vi "ENPH 354 Assignment 2 - Q3 .vi"() -> ()   [LabVIEW 2021]
panel:
  out "Top Right":bool
  out "Top":bool
  out "Top Left":bool
  out "Middle":bool
  out "Bottom Right":bool
  out "Bottom Left":bool
  out "Bottom":bool
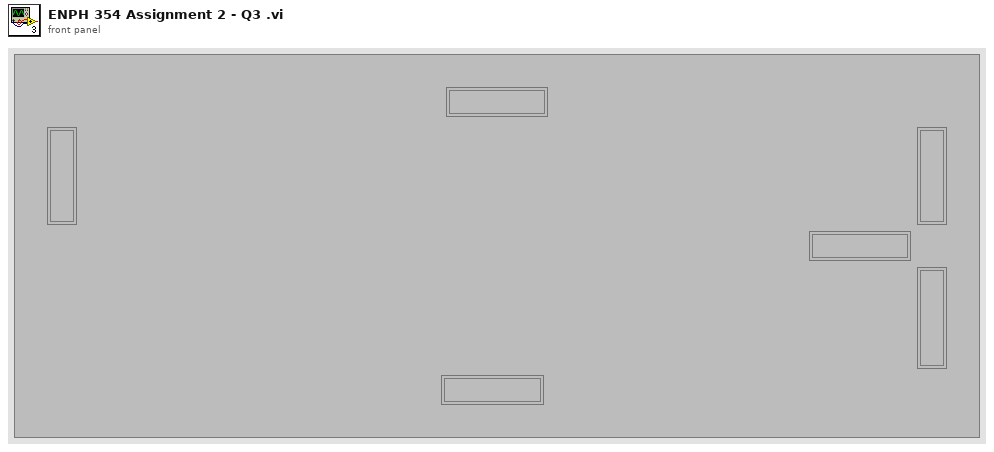
[diagram p1: front panel]
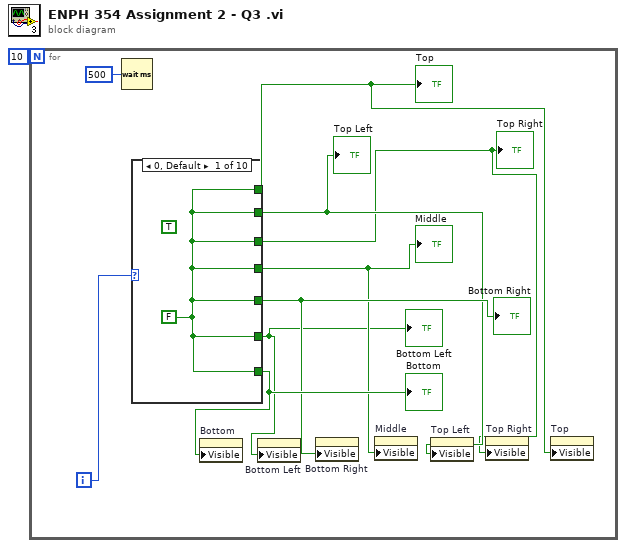
[diagram p0: block diagram]
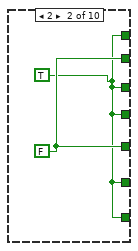
[diagram p2: hidden frame]
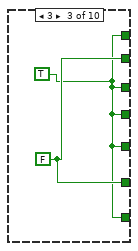
[diagram p3: hidden frame]
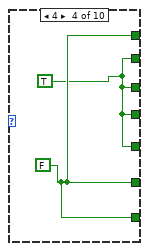
[diagram p4: hidden frame]
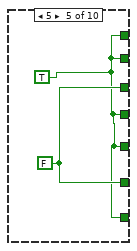
[diagram p5: hidden frame]
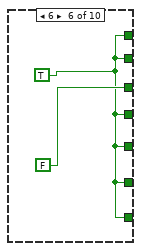
[diagram p6: hidden frame]
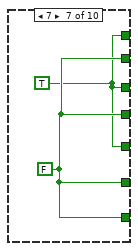
[diagram p7: hidden frame]
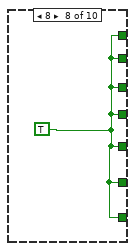
[diagram p8: hidden frame]
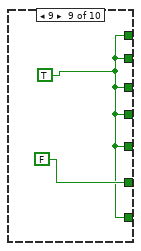
[diagram p9: hidden frame]
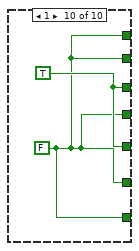
[diagram p10: hidden frame]
diagram:
  n1 = for {
    N: 10 -> [_]
    i -> [w9]
    n2 = Wait (ms)(milliseconds to wait=u32 500) -> ()  [unwired: 1 out]
    n3 = case shown="0, Default" w9 {
      tunnel: [w11 w12 w14 w17 w18 w20 w22 w24 w25 w27] -> w3
      tunnel: [w11 w13 w15 w16 w18 w20 w23 w24 w25 w27] -> w5
      tunnel: [w11 w12 w14 w16 w19 FALSE w22 w24 w25 w28] -> w4
      tunnel: [w11 w12 w14 w16 w18 w20 w23 w24 w25 w27] -> w6
      tunnel: [w11 w13 w14 w16 w18 w20 w22 w24 w25 w28] -> w7
      tunnel: [w11 w12 w15 w17 w19 w20 w23 w24 FALSE w27] -> w2
      tunnel: [w11 w12 w14 w17 w18 w20 w23 w24 w25 w27] -> w8
      frame 0, Default {
        w11 = FALSE
        (unwired) TRUE
      }
      frame 2 {
        w13 = FALSE
        w12 = TRUE
      }
      frame 3 {
        w15 = FALSE
        w14 = TRUE
      }
      frame 4 {
        w17 = FALSE
        w16 = TRUE
      }
      frame 5 {
        w19 = FALSE
        w18 = TRUE
      }
      frame 6 {
        w20 = TRUE
      }
      frame 7 {
        w23 = FALSE
        w22 = TRUE
      }
      frame 8 {
        w24 = TRUE
      }
      frame 9 {
        w25 = TRUE
      }
      frame 1 {
        w27 = FALSE
        w28 = TRUE
      }
    }
    "Bottom" <- w8
    "Middle" <- w6
    "Top Left" <- w5
    "Top" <- w3
    "Top Right" <- w4
    "Bottom Left" <- w2
    "Bottom Right" <- w7
    n4 = property on="Bottom" class="Bool (strict)"("Visible"=w8) -> ()  [unwired: 2 in, 2 out]
    n5 = property on="Bottom Left" class="Bool (strict)"("Visible"=w2) -> ()  [unwired: 2 in, 2 out]
    n6 = property on="Bottom Right" class="Bool (strict)"("Visible"=w7) -> ()  [unwired: 2 in, 2 out]
    n7 = property on="Middle" class="Bool (strict)"("Visible"=w6) -> ()  [unwired: 2 in, 2 out]
    n8 = property on="Top Left" class="Bool (strict)"("Visible"=w5) -> ()  [unwired: 2 in, 2 out]
    n9 = property on="Top Right" class="Bool (strict)"("Visible"=w4) -> ()  [unwired: 2 in, 2 out]
    n10 = property on="Top" class="Bool (strict)"("Visible"=w3) -> ()  [unwired: 2 in, 2 out]
  }
